vi "Read Rate A (GPM).vi"(8 "error out":errorcluster, 11 "VISA resource name out":refnum<visa-resource-name>) -> (0 "error IO":errorcluster, 2 "GPM":dbl, 3 "VISA resource  out":refnum<visa-resource-name>)   [LabVIEW 2010, in "FEM-03.lvlib"]
uses:
  FEM-03.lvlib
  Private/Controls/Variable List.ctl
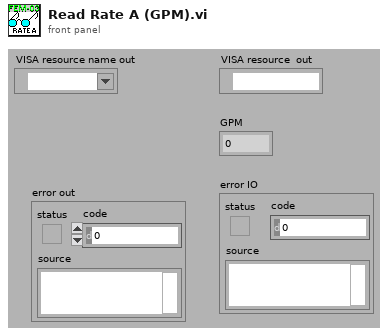
[diagram p1: front panel]
types:
  T1 = typedef "FEM-03.lvlib/Variable List.ctl" = enum16{"Rate A (PL)", "Rate A (GT)", "Job Total A", "Grand Total A", "A-KFR for Rate", "A-KFR decimal point location", "A-KFT for Total", "A-KFT decimal point location ", "A-Rate Engineering Units", "A-Total Engineering units", "A-Flow Direction", "Rate B (PL)", "Rate B (GT)", "Job Total B", "Grand Total B", "B-KFR for Rate", "B-KFR deciminal point location", "B-Rate Engineering units", "B-KFT for Total", "B-KFT decimal point location", "B-Total Engineering units", "Limit 1 Mode", "Limit1", "Margin 1 for rate limit", "Limit 2 Mode", "Limit2", "Margin 2 for rate limit", "Milli-amps Offset", "Milli-amps Out", "Analog Out Mode", "Serial Speed", "Unit Number", "Serial RESET TOTAL", "Update EEPROM", "Relay Override", "FORCE mA Output"}
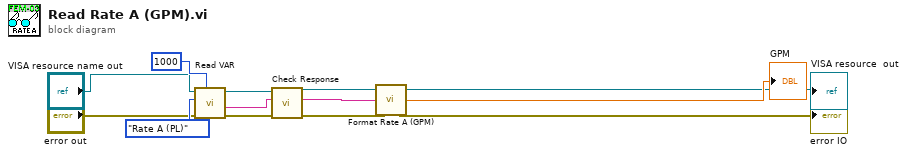
[diagram p0: block diagram]
diagram:
  n1 = call "Read VAR.vi"("Timeout (ms)"=u32 1000, "error in"="error out", "Variable to Read"=Variable_List."Rate A (PL)", "VISA resource name"="VISA resource name out") -> ("error out"=w7:errorcluster, "Read Buffer"=w5:string, "VISA resource name out"=w6:refnum<visa-resource-name>)  [unwired: 5 in]
  n2 = call "Check Response.vi"("Error In"=w7, "Read Buffer"=w5, "VISA resource"=w6) -> ("error out"=w9:errorcluster, "Filtered Response"=w8:string, "VISA resource  out"=w10:refnum<visa-resource-name>)  [unwired: 6 in]
  n3 = call "Format Rate A (GPM).vi"("error out"=w9, "Filtered Response"=w8, "VISA resource  in"=w10) -> ("error IO"=→"error IO":errorcluster, "GPM"=→"GPM":dbl, "VISA resource  out"=→"VISA resource  out":refnum<visa-resource-name>)
